vi "Main.vi"   [LabVIEW 2011]
types:
  T1 = typedef "WPI_DriverStationRobotMode.ctl" = enum16{"Autonomous Disabled", "Autonomous Enabled", "Teleop Disabled", "Teleop Enabled", "Timeout", "Finish"}
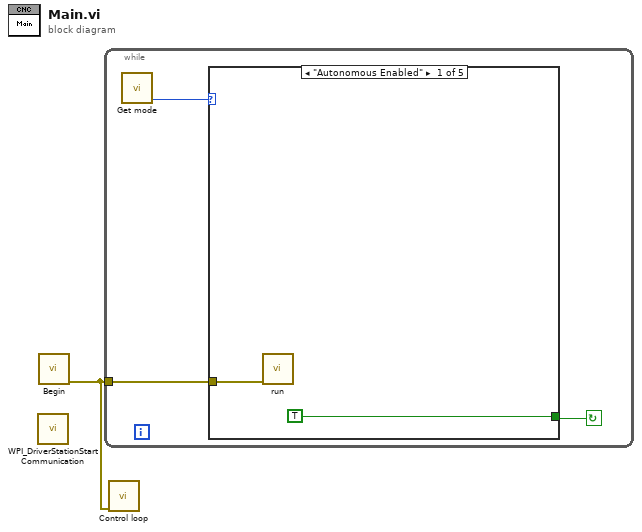
[diagram p0: block diagram]
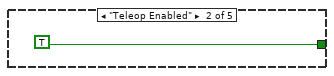
[diagram p2: hidden frame]
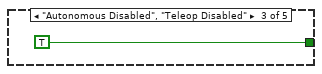
[diagram p3: hidden frame]
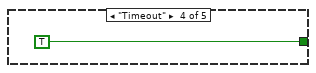
[diagram p4: hidden frame]
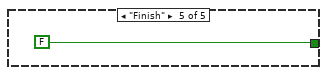
[diagram p5: hidden frame]
diagram:
  n1 = call <vilib>:"WPI_DriverStationStart Communication.vi"() -> ()  [unwired: 12 in]
  n2 = call "Begin.vi"() -> ("error out"=w1:errorcluster)  [unwired: 11 in]
  n3 = while {
    tunnel: w1 -> [w4]
    stop <- w2 continue-if-true
    n4 = call "Get mode.vi"() -> ("Robot Mode"=w3:T1)  [unwired: 11 in]
    n5 = case shown="\"Autonomous Enabled\"" w3 {
      tunnel: [TRUE TRUE TRUE TRUE FALSE] -> w2
      tunnel: w4 -> [w5 _ _ _ _]
      frame "Autonomous Enabled" {
        n6 = call "run.vi"("error in (no error)"=w5) -> ()  [unwired: 10 in, 1 out]
      }
      frame "Teleop Enabled" {
      }
      frame "Autonomous Disabled", "Teleop Disabled" {
      }
      frame "Timeout" {
      }
      frame "Finish" {
      }
    }
  }
  n7 = call "Control loop.vi"("error in (no error)"=w1) -> ()  [unwired: 11 in]
